vi "Sandbox 5 - Move a VI from one virtual folder to another.vi"() -> ()   [LabVIEW 2022 SP3]
uses:
  DFS Output (cluster).ctl
  40687720-449f-4ff4-8850-91d26a6e7aa5.vi
panel:
  out "Type String":string
  out "Name":string
  out "Project Names":string[](array[string])
  out "Number of projects":i32
  out "Project:Projects[]":refnum<vi>[](array[refnum])
  out "Search Output":T1
  out "Virtual Folder Path (index 0 is top-level folder)":string[](array[string])
  out "Destination Folder Found?":bool
  out "Destination Folder Refnum":refnum<vi>
  out "Number of owned items":i32
  in  "Destination Folder":string="Folder1"
  out "Number of folders":i32
  out "error out":errorcluster
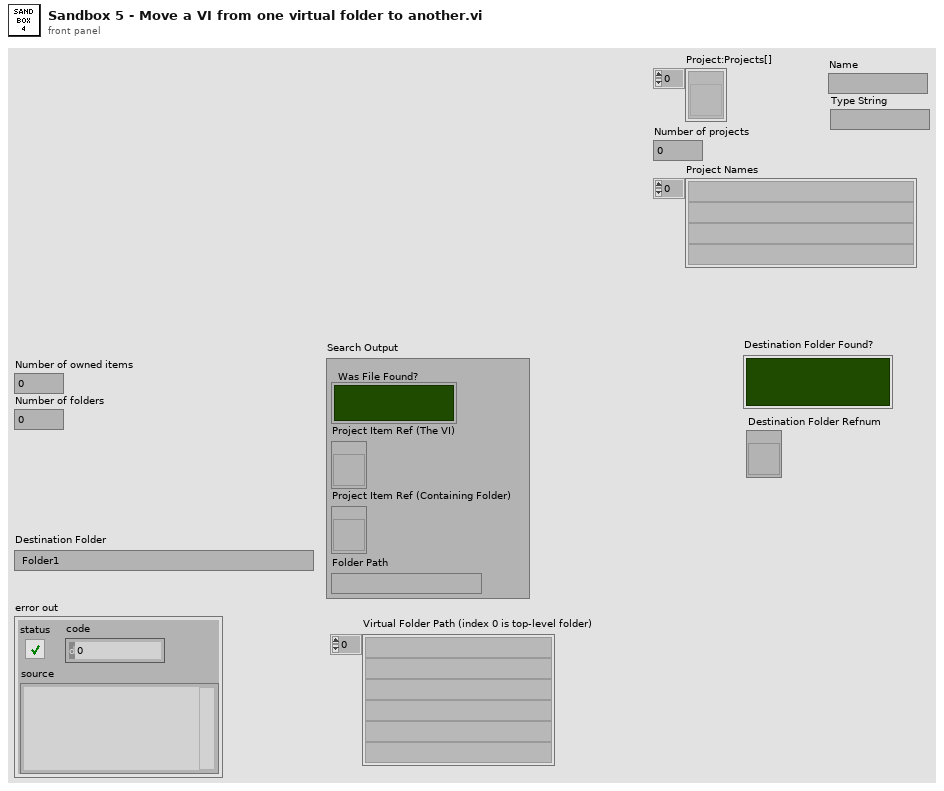
[diagram p1: front panel]
types:
  T1 = typedef "DFS Output (cluster).ctl" = cluster{"Was File Found?":bool, "Project Item Ref (The VI)":refnum<vi>, "Project Item Ref (Containing Folder)":refnum<vi>, "Folder Path":string}
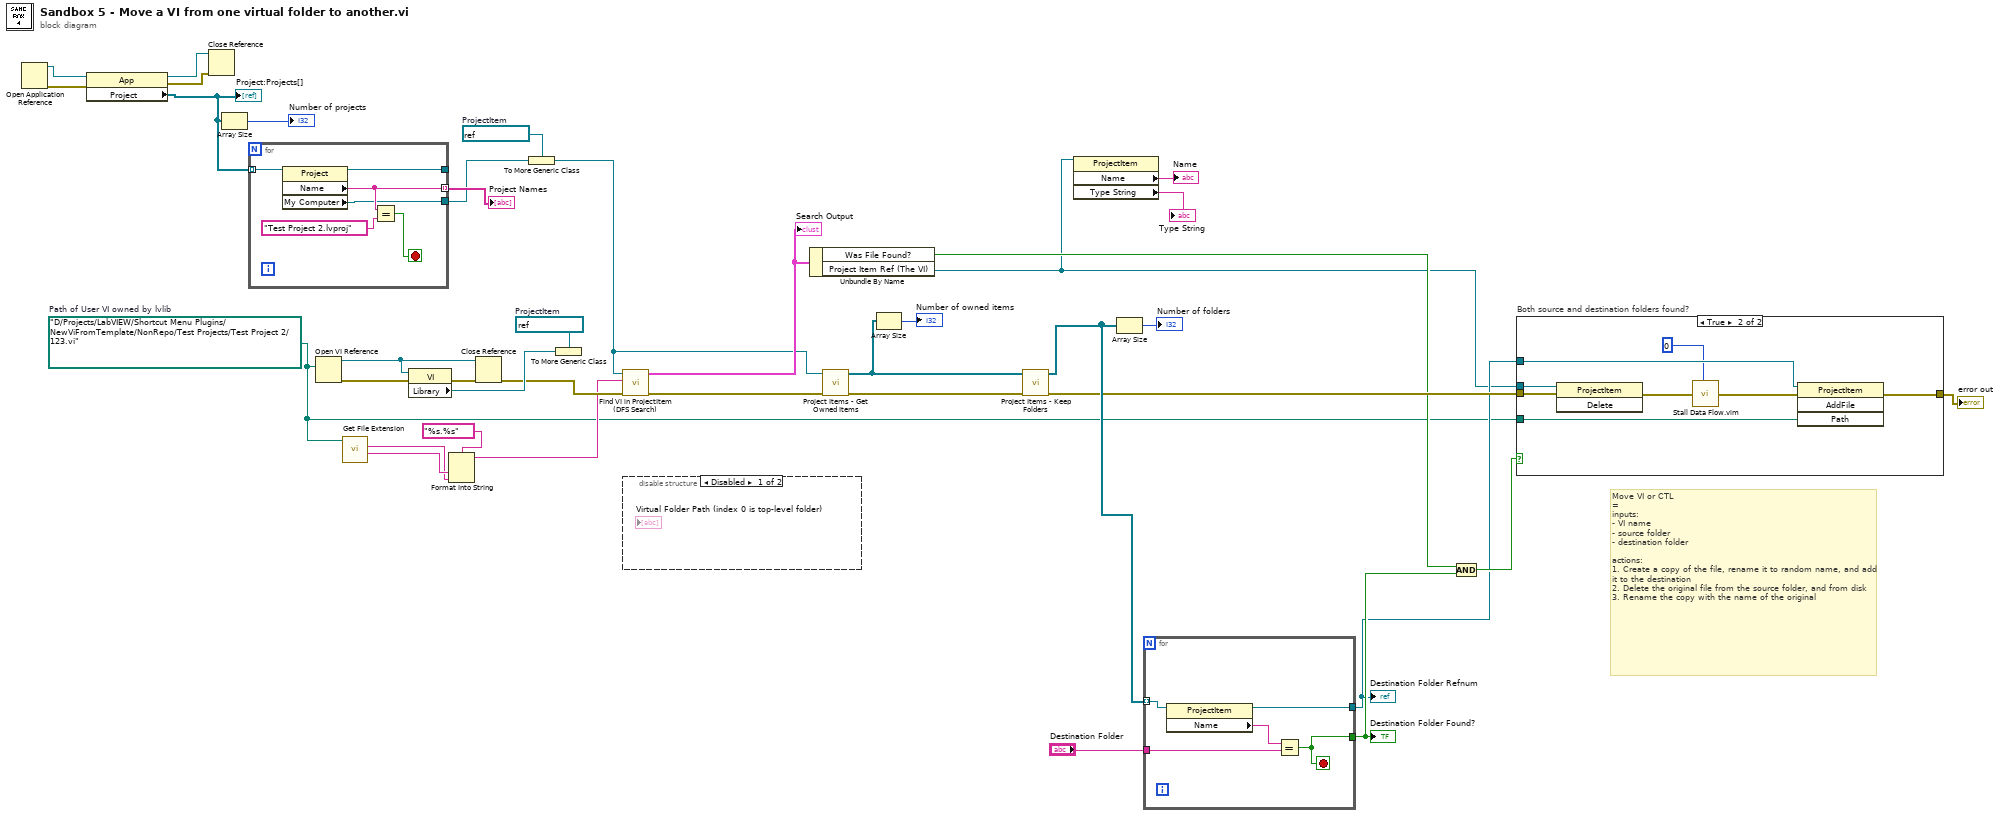
[diagram p0: block diagram]
diagram:
  w6 = refnum<vi> refnum  # ProjectItem
  w36 = refnum<vi> refnum  # ProjectItem
  w14 = path "D:/Projects/LabVIEW/Shortcut Menu Plugins/NewViFromTemplate/NonRepo/Test Projects/Test Project 2/123.vi"  # Path of User VI owned by lvlib
  # "Move VI or CTL\n=\ninputs:\n- VI name\n- source folder\n- destination folder\n\nactions:\n1. Create a copy of the file, rename it to random name, and add it to the destination\n2. Delete the original file from the source folder, and from disk\n3. Rename the copy with the name of the original"
  n1 = Open Application Reference() -> (0:w12:errorcluster, 3:w13:refnum<vi>)  [unwired: 4 in]
  n2 = property class="App"(reference=w13, error in=w12) -> (reference out=w7:refnum<vi>, error out=w8:errorcluster, "Project"=w10:refnum<vi>[])
  "Project:Projects[]" <- w10
  n3 = Close Reference(reference=w7, error in (no error)=w8) -> ()  [unwired: 1 out]
  n4 = Array Size(array=w10) -> (size(s)=→"Number of projects":i32)
  n5 = for {
    tunnel: w10 -> [w44] mode=indexing
    tunnel: [w42] -> w9 mode=indexing
    tunnel: [w40] -> _
    tunnel: [w39] -> w5
    stop <- w41 stop-if-true
    n6 = property class="Project"(reference=w44) -> (reference out=w40:refnum<vi>, "Name"=w42:string, "My Computer"=w39:refnum<vi>)  [unwired: 1 in, 1 out]
    n7 = Equal?(x=w42, y="Test Project 2.lvproj" ("Name")) -> (x = y?=w41:bool)
  }
  "Project Names" <- w9
  n8 = Open VI Reference(vi path=w14) -> (vi reference=w28:refnum<vi>, error out=w38:errorcluster)  [unwired: 5 in]
  n9 = call <vilib>:"Get File Extension.vi"("file"=w14) -> ("filename without extension"=w19:string, "lowercase file extension"=w18:string)  [unwired: 6 in, 3 out]
  n10 = property class="VI"(reference=w28, error in=w38) -> (error out=w34:errorcluster, "Library"=w35:refnum<vi>)  [unwired: 1 out]
  n11 = Format Into String(format string="%s.%s", w19, w18) -> (resulting string=w20:string)  [unwired: 2 in, 1 out]
  n12 = Close Reference(reference=w28, error in (no error)=w34) -> (error out=w23:errorcluster)
  n13 = To More Generic Class(target class=w6, reference=w5) -> (generic class reference=w4:refnum<vi>)
  n14 = To More Generic Class(target class=w36, reference=w35) -> ()  [unwired: 1 out]
  n15 = call "Find VI in ProjectItem (DFS Search).vi"("Error In"=w23, "VI Filename (including extension)"=w20, "Project Item Ref"=w4) -> ("Error Out"=w22:errorcluster, "Search Output"=w17:T1)  [unwired: 7 in]
  "Search Output" <- w17
  n16 = disable-structure shown="Disabled" {
    frame Disabled {
    }
    frame Enabled {
    }
  }
  n17 = Unbundle By Name(w17) -> ("Was File Found?"=w16:bool, "Project Item Ref (The VI)"=w3:refnum<vi>)
  n18 = call "Project Items - Get Owned Items.vi"("Error In"=w22, "Project Item"=w4) -> ("Error Out"=w33:errorcluster, "Owned Items"=w31:refnum<vi>[])  [unwired: 8 in]
  n19 = Array Size(array=w31) -> (size(s)=→"Number of owned items":i32)
  n20 = call "Project Items - Keep Folders.vi"("Error In"=w33, "Project Items"=w31) -> ("Error Out"=w27:errorcluster, "Project Items (Folders)"=w30:refnum<vi>[])  [unwired: 8 in]
  n21 = property class="ProjectItem"(reference=w3) -> ("Name"=→"Name":string, "Type String"=→"Type String":string)  [unwired: 1 in, 2 out]
  n22 = Array Size(array=w30) -> (size(s)=→"Number of folders":i32)
  n23 = for {
    tunnel: w30 -> [w49] mode=indexing
    tunnel: "Destination Folder" -> [w47]
    tunnel: [w46] -> w15
    tunnel: [w45] -> w25
    stop <- w45 stop-if-true
    n24 = property class="ProjectItem"(reference=w49) -> (reference out=w46:refnum<vi>, "Name"=w48:string)  [unwired: 1 in, 1 out]
    n25 = Equal?(x=w48, y=w47) -> (x = y?=w45:bool)
  }
  "Destination Folder Refnum" <- w15
  "Destination Folder Found?" <- w25
  n26 = Compound Arithmetic op=AND(w16, w25) -> (w24:bool)
  n27 = case "Both source and destination folders found?" shown="True" w24 {
    tunnel: w27 -> [w50 w58]
    tunnel: [w50 w57] -> w26
    tunnel: w3 -> [_ w55]
    tunnel: w15 -> [_ w54]
    tunnel: w14 -> [_ w53]
    frame False {
    }
    frame True {
      n28 = invoke class="ProjectItem" method="Delete"(reference=w55, error in=w58) -> (error out=w56:errorcluster)  [unwired: 1 in, 2 out]
      n29 = call "Stall Data Flow.vim"("value in"=w56, "milliseconds to wait"=u32 0) -> ("value out"=w52:errorcluster)  [unwired: 1 out]
      n30 = invoke class="ProjectItem" method="AddFile"(reference=w54, error in=w52, "Path"=w53) -> (error out=w57:errorcluster)  [unwired: 1 in, 3 out]
    }
  }
  "error out" <- w26
